vi "Steer_Utilitiy.vi"(4 "right":bool, 6 "left":bool, 7 "increment":i16, 11 "Array":bool[](array[boolean])) -> (0 "Turn Signal":i8, 3 "steer":i16)   [LabVIEW 2015]
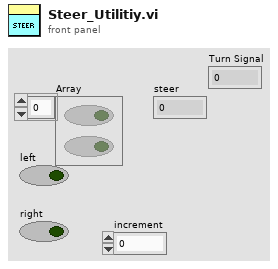
[diagram p1: front panel]
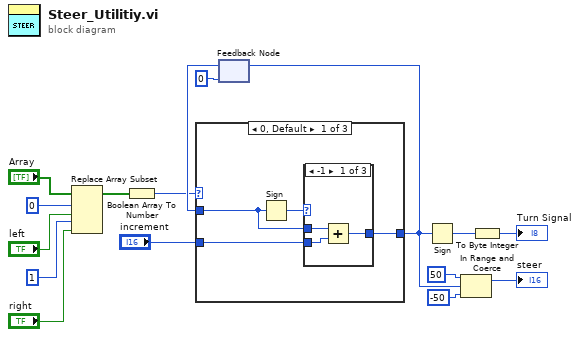
[diagram p0: block diagram]
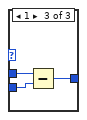
[diagram p3: hidden frame]
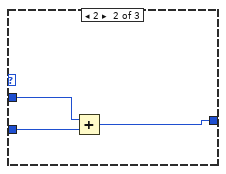
[diagram p4: hidden frame]
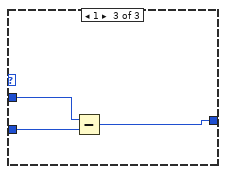
[diagram p5: hidden frame]
diagram:
  n1 = Replace Array Subset(array="Array", new element #1="left", index #1=0 ("index"), new element #2="right", index #2=1 ("index")) -> (w11:bool[])
  n2 = Boolean Array To Number(Boolean array=w11) -> (number=w12:u32)
  n3 = feedback #1(i16 0 ("upper limit")) -> (w13:i16)
  n4 = case shown="0, Default" w12 {
    tunnel: [w19 w29 w32] -> w3
    tunnel: w13 -> [w18 w30 w33]
    tunnel: "increment" -> [w17 w28 w31]
    frame 0, Default {
      n5 = Sign(1:w18) -> (0:w20:i16)
      n6 = case shown="-1" w20 {
        tunnel: [w22 w24 w27] -> w19
        tunnel: w18 -> [w23 w24 w26]
        tunnel: w17 -> [w21 _ w25]
        frame -1 {
          n7 = Add(x=w23, y=w21) -> (x+y=w22:i16)
        }
        frame 0, Default {
        }
        frame 1 {
          n8 = Subtract(x=w26, y=w25) -> (x-y=w27:i16)
        }
      }
    }
    frame 2 {
      n9 = Add(x=w30, y=w28) -> (x+y=w29:i16)
    }
    frame 1 {
      n10 = Subtract(x=w33, y=w31) -> (x-y=w32:i16)
    }
  }
  n11 = feedback-in #1(w3) -> ()
  n12 = Sign(1:w3) -> (0:w2:i16)
  n13 = In Range and Coerce(upper limit=i16 50, x=w3, lower limit=i16 -50) -> (coerced(x)=→"steer":i16)  [unwired: 1 out]
  n14 = To Byte Integer(number=w2) -> (8bit integer=→"Turn Signal":i8)
